vi "Account FGV.vi"(7 "Account Methods":T1, 8 "error in":errorcluster, 11 "Amount":dbl) -> (0 "error out":errorcluster, 3 "Account Balance":dbl)   [LabVIEW 2014]
uses:
  Account Methods.ctl
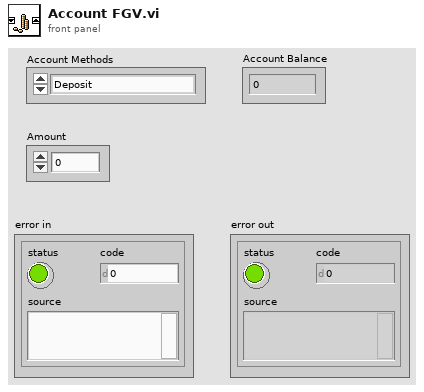
[diagram p1: front panel]
types:
  T1 = typedef "Account Methods.ctl" = enum16{"Deposit", "Withdraw", "Get Balance", "Clear Balance"}
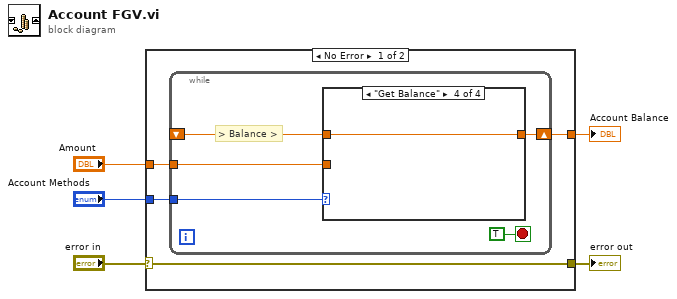
[diagram p0: block diagram]
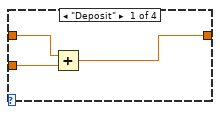
[diagram p2: hidden frame]
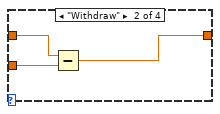
[diagram p3: hidden frame]
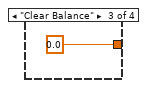
[diagram p4: hidden frame]
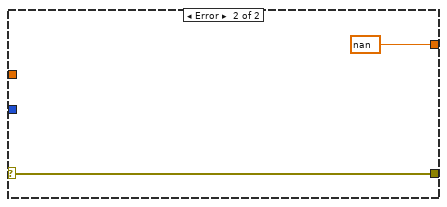
[diagram p5: hidden frame]
diagram:
  n1 = case shown="No Error" "error in" {
    selector: "error in" -> [w6 w24]
    tunnel: "Amount" -> [w9 _]
    tunnel: "Account Methods" -> [w8 _]
    tunnel: [w7 sgl nan] -> w3
    tunnel: [w6 w24] -> w1
    frame No Error {
      n2 = while {
        shift-right: [w12] -> w7
        shift-left: _ -> [w13]
        tunnel: w9 -> [w11]
        tunnel: w8 -> [w10]
        stop <- TRUE stop-if-true
        # "> Balance >"
        n3 = case shown="\"Get Balance\"" w10 {
          tunnel: w11 -> [w17 w20 _ _]
          tunnel: w13 -> [w16 w19 _ w22]
          tunnel: [w15 w18 0.0 w22] -> w12
          frame "Deposit" {
            n4 = Add(x=w16, y=w17) -> (x+y=w15:dbl)
          }
          frame "Withdraw" {
            n5 = Subtract(x=w19, y=w20) -> (x-y=w18:dbl)
          }
          frame "Clear Balance" {
          }
          frame "Get Balance" {
          }
        }
      }
    }
    frame Error {
    }
  }
  "error out" <- w1
  "Account Balance" <- w3
